vi "Get Selected Index Terminal from Unbundler (by oneof name).vi"(8 "error in (no error)":errorcluster, 10 "Oneof Container Name":string, 11 "Unbundler in":refnum<vi>) -> (0 "error out":errorcluster, 1 "Found?":bool, 2 "Terminal Refnum":refnum<vi>, 3 "Unbundler out":refnum<vi>)   [LabVIEW 2019, in "gRPC Template Creation Utility.lvlib"]
uses:
  gRPC Template Creation Utility.lvlib
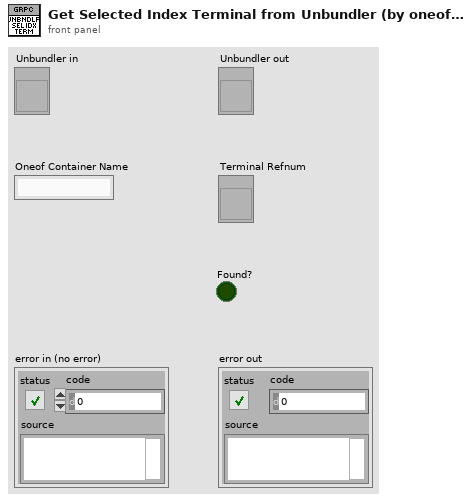
[diagram p1: front panel]
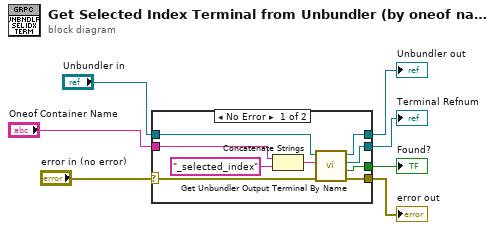
[diagram p0: block diagram]
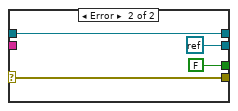
[diagram p2: hidden frame]
diagram:
  n1 = case shown="No Error" "error in (no error)" {
    selector: "error in (no error)" -> [w8 w20]
    tunnel: "Unbundler in" -> [w16 w19]
    tunnel: "Oneof Container Name" -> [w13 _]
    tunnel: [w12 w20] -> w5
    tunnel: [w11 FALSE ("Found?")] -> w4
    tunnel: [w10 refnum<k0> refnum] -> w3
    tunnel: [w9 w19] -> w2
    frame No Error {
      n2 = Concatenate Strings(w13, "_selected_index" ("string")) -> (w14:string)
      n3 = call "Get Unbundler Output Terminal By Name.vi"("error in (no error)"=w8, "Terminal name"=w14, "Unbundler in"=w16) -> ("error out"=w12:errorcluster, "Found?"=w11:bool, "Terminal Refnum"=w10:refnum<vi>, "Unbundler out"=w9:refnum<vi>)  [unwired: 5 in]
    }
    frame Error {
    }
  }
  "error out" <- w5
  "Found?" <- w4
  "Terminal Refnum" <- w3
  "Unbundler out" <- w2
